vi "run.vi"(8 "error in (no error)":errorcluster, 9 "deviceDataBase":refnum<class "deviceDataBase.lvclass">, 10 "HWControllerEvents":refnum<class "HWControllerEvents.lvclass">, 11 "Compiler in":refnum<class "Compiler.lvclass">) -> (0 "error out":errorcluster, 3 "Compiler out":refnum<class "Compiler.lvclass">)   [LabVIEW 2009, in "Compiler.lvlib" / "Compiler.lvclass"]
uses:
  Compiler.lvclass
  Hal/HWController/HWControllerEvents/HWControllerEvents.lvclass
  DatabaseHelpers/DbConnection/DeviceDataBase/deviceDataBase.lvclass
  Filing/FileSystem/FileSystem.lvclass
  Compiler.lvclass/Compiler.ctl
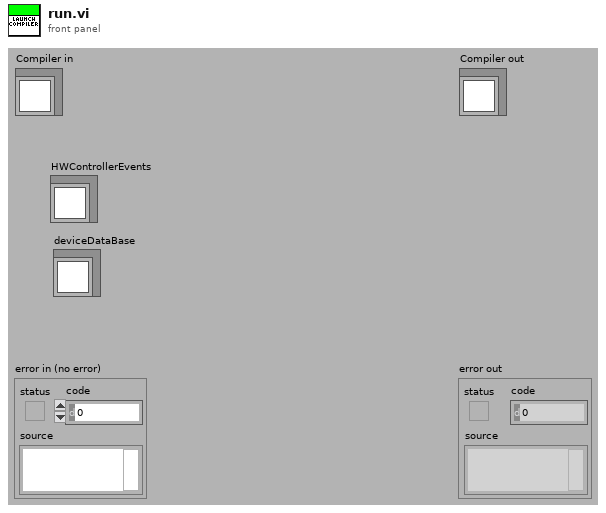
[diagram p1: front panel]
types:
  T1 = enum32{"Invalid", "Standard", "Closed", "Hidden", "Minimized", "Maximized"}
  T2 = enum32{"Bad", "Idle", "Run top level", "Running"}
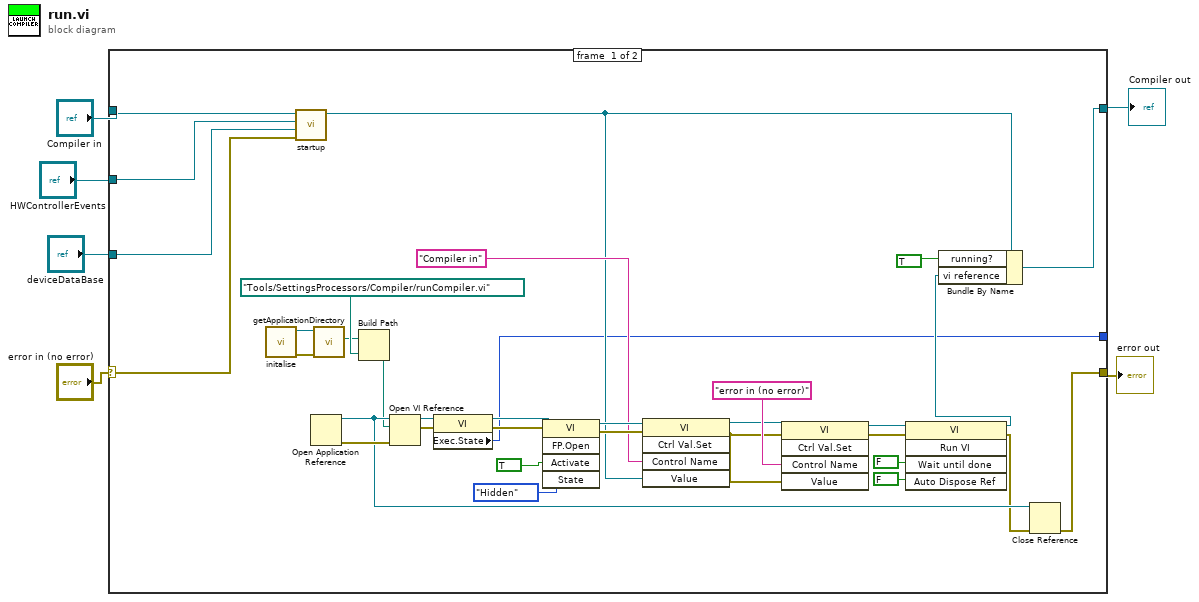
[diagram p0: block diagram]
diagram:
  n1 = case shown="No Error" "error in (no error)" {
    selector: "error in (no error)" -> [w19 w41]
    tunnel: [w31 w41] -> w4
    tunnel: [w11 w42] -> w5
    tunnel: "Compiler in" -> [w22 w42]
    tunnel: "HWControllerEvents" -> [w21 _]
    tunnel: "deviceDataBase" -> [w20 _]
    tunnel: [w7 _] -> _
    frame #0 {
      n2 = call "initalise.vi"() -> ("error out"=w17:errorcluster, "FileSystem out"=w18:refnum<class "FileSystem.lvclass">)  [unwired: 10 in]
      n3 = call "startup.vi"("error in (no error)"=w19, "deviceDataBase"=w20, "HWControllerEvents"=w21, "Compiler in"=w22) -> ("Compiler out"=w12:refnum<class "Compiler.lvclass">)  [unwired: 6 in, 1 out]
      n4 = Open Application Reference() -> (0:w37:errorcluster, 3:w33:refnum<vi>)  [unwired: 4 in]
      n5 = call-dynamic "getApplicationDirectory.vi"("error in (no error)"=w17, "FileSystem.lvclass in"=w18) -> ("ApplicationDirectory"=w15:path)  [unwired: 7 in, 2 out]
      n6 = Build Path(base path=w15, name or relative path=path "Tools/SettingsProcessors/Compiler/runCompiler.vi" ("vi path")) -> (appended path=w14:path)
      n7 = Open VI Reference(application reference (local)=w33, vi path=w14, error in (no error)=w37) -> (vi reference=w28:refnum<vi>, error out=w8:errorcluster)  [unwired: 3 in]
      n8 = property class="VI"(reference=w28, error in=w8) -> (reference out=w10:refnum<vi>, error out=w9:errorcluster, "Exec.State"=w7:T2)
      n9 = invoke class="VI" method="FP.Open"(reference=w10, error in=w9, "Activate"=TRUE, "State"=T1."Hidden") -> (reference out=w27:refnum<vi>, error out=w26:errorcluster)  [unwired: 1 in, 3 out]
      n10 = invoke class="VI" method="Ctrl Val.Set"(reference=w27, error in=w26, "Control Name"="Compiler in", "Value"=w12) -> (reference out=w36:refnum<vi>, error out=w35:errorcluster)  [unwired: 1 in, 3 out]
      n11 = invoke class="VI" method="Ctrl Val.Set"(reference=w36, error in=w35, "Control Name"="error in (no error)", "Value"=w35) -> (reference out=w30:refnum<vi>, error out=w29:errorcluster)  [unwired: 1 in, 3 out]
      n12 = invoke class="VI" method="Run VI"(reference=w30, error in=w29, "Wait until done"=FALSE, "Auto Dispose Ref"=FALSE) -> (reference out=w24:refnum<vi>, error out=w32:errorcluster)  [unwired: 1 in, 3 out]
      n13 = Bundle By Name(cluster=w12, "running?"=TRUE, "vi reference"=w24) -> (w11:refnum<class "Compiler.lvclass">)
      n14 = Close Reference(reference=w33, error in (no error)=w32) -> (error out=w31:errorcluster)
    }
    frame #1 {
    }
  }
  "error out" <- w4
  "Compiler out" <- w5
